vi "Translator.File.Read.FP.vi"(4 "progressbar2":refnum<vi>, 5 "init":bool, 6 "progressbar1":refnum<vi>, 7 "Message":refnum<vi>, 8 "error in":errorcluster, 9 "font name":string, 11 "Translation file":path=path "D:/PL_0125_Sapphire_Automation_branches/SOFTWARE_v1.1-Translation/settings/Translation-Chinese.ini") -> (0 "error out":errorcluster)   [LabVIEW 2016]
uses:
  Translator.Message.ctl
  Translator.Control.Fglb.Action.vi
  Translator.FormatMessage.vi
  Translator.Global.vi
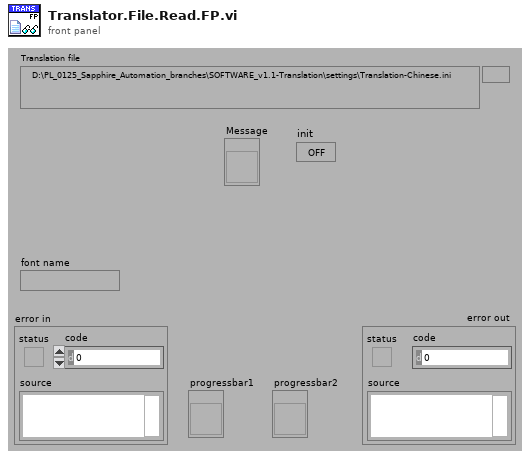
[diagram p1: front panel]
types:
  T1 = typedef "Translator.Message.ctl" = enum16{"-", "Event confirmed", "Log out", "Log in", "Shutdown", "Cancel", "Start", "Begin time", "End time", "Duration", "Service Mode", "Ignore Results", "Serial Format", "On", "Off", "OK", "NOK", "NOK %s", "Home", "Work", "Close", "Open", "In progress...", "Missing", "Empty", "Hardware failure", "Initial", "Default", "Total", "Out of range", "Free disk space is below 1GB - contact technician", "Error %d >> %s", "Error %d >> %s >> %s", "Msg %d >> %s", "Laser msg %d %s", "Laser cmd error %s %d", "Laser cmd failed %s", "Laser cmd warning %s", "Laser disconnected", "Laser status %s", "Laser already started", "Laser job unkonwn %s", "Laser job missing %s", "Laser job select failure %s", "Unable to start laser printing (%s)", "Unable to stop laser printing (%s)", "Laser marking aborted", "Laser marking timeout", "Unable to reset Laser Interlock (%s)", "Unable to trigger Laser. Laser not ready (%s)", "Laser job '%s' coordinates not configured", "Starting %s", "Quitting %s", "Configured", "Initializing", "Quitting", "Loading", "Loaded %d results", "Loaded %d events", "Running", "Stopped", "Summary", "Laser", "Do you want to continue?", "Do you want to delete the configuration?", "The configuration is being used by an order. Unable to delete!", "Press confirm button", "Station is not based. Do you want to exit?", "Station requires changeover. Do you want to run the test?", "Test options are not set as default. Do you want to continue?", "Formatting of WabcoNo is disabled. Do you want to continue?", "Product not detected. Do you want to continue?", "Product scan failed. Do you want to continue?", "Calibration", "Log out?", "System", "All", "IDLE", "Translating...%s", "Not found", "Alarm %s", "Run", "Skip", "Abort", "Repeat", "Please wait...", "Database disconnected", "Database disconnected - changeover disabled!", "Login to database successful", "Login to database failed: %d; %s", "Unable to check the product status of reference %d - database disconnected", "Unable to set the product status of reference %d - database disconnected", "Variant file backup %s", "Read variant (%s)", "Result", "Station armed!", "Station requires changeover!", "Select reference number...", "EMERGENCY BUTTON - press Control button", "EMERGENCY DOOR - press Control button", "Resetting Emergency...", "Unable to reset safety circuit - Emergency Button pressed", "Unable to reset safety circuit - Emergency Side Door open", "Station not based", "Station based", "Station not empty", "Station basing...", "No order", "Press Start to begin new order", "Scanning new order", "Order NOK. Correct or scan again", "Order OK. Press Accept", "Order ready", "Revolver incorrect", "Fork incorrect", "Revolver missing", "Revolver empty", "Container missing", "Offline results", "Offline statistics", "Updating statistics %.1f %%", "DMC Configurator", "Door open", "Close the front door", "Press start button", "Done. Open the front door", "Running...", "Running...%.1f %%", "Pause %s", "Pause %s. NOK container missing", "Pause %s. OK container missing", "Pause %s. Revolver empty", "Pause %s. Revolver missing", "Pause %s. Revolver incorrect", "Pause %s. Fork missing", "Pause %s. Fork incorrect", "Pause %s. Too many failures", "Pause %s. Unloading failure", "Pause %s. One slot is not working", "Pause %s. Part order is done. Empty OK container", "Pause %s. Unable to move product to slot", "Pause %s. Unable to move back product pusher", "Pause %s. Unable to lift product", "Pause %s. Unable to move back product lifter", "Pause %s. Unable to move product arm to Work", "Pause %s. Unable to move product arm to NOK", "Pause %s. Unable to move product arm to OK", "Pause %s. Unable to unsuck the NOK product", "Pause %s. Unable to drop the NOK product", "Pause %s. Product OK missing", "Pause %s. Unable to unsuck the OK product", "Pause %s. Unable to drop the OK product", "Stopping...", "File '%s' is missing", "File '%s' is broken", "File '%s' is running", "Log file started (%s)", "Log file ended (%s)", "Log file stopped (%s)", "Log file ignored (%s)", "Log file exported (%s)", "Log file export failed (%s)", "Wrong serial number in log file", "Wrong reference number in log file", "Test steps are missing", "%s = %.3f", "Process param '%s' not found in DB", "Process param '%s' wrong order", "Process param '%s' value %.3f out of limits (%.3f; %.3f)", "Step%d param '%s' not found in DB", "Step%d param '%s' wrong order", "Step%d param '%s' value %.3f out of limits (%.3f; %.3f)", "Step%d EV '%s' not found in DB", "Step%d EV '%s' wrong order", "\"%s\" not found in DB", "\"%s\" wrong order", "\"%s\" value %.3f out of limits (%.3f; %.3f)", "\"%s\" not found in software", "Process init (%s)", "Process started", "Process restarted", "Process run", "Process done", "Process done - remove OK container", "Process aborted", "Process aborted at work", "Process aborted at home", "Process error", "Process error at home", "Process error at work", "Process close", "Process pause", "Process continue", "Process door open", "Process door close", "Process pause at slot %s due to %s", "Select plate from the order to process", "Do you want to start the process?", "Do you want to continue the process?", "There is unfinished order. Do you want to put the new order?", "Product %s %d OK", "Product %s %d NOK", "Unable to unload the slot %s. Product missing in the slot", "Unable to unload the slot %s. Product already in the arm", "Unable to accept the product as OK. Product missing in slot %s", "Unable to accept the product as OK. Product could not drop into the container at slot %s", "Unable to accept the product as NOK. Product could not drop into the container at slot %s", "Scan failed. Error %s", "Scan failed. Scanner disconnected", "Scan failed. Wrong Wabco number %d, limit (%d,%d)", "Scan failed. Wrong serial number %d, limit (%d,%d)", "Scan failed. Wrong date %d, limit (%d,%d)", "Scan failed. Wrong product wabco number %d (expected %d)", "Scan failed. Wrong product serial number %d (expected > 0)", "Scan OK %s", "Scan failed. Unable to determine table position (%s)", "Scan failed. Timeout", "Tune failed. Scanner disconnected", "Tune failed. Timeout", "%s = %d", "%s = %d->%d", "Unable to set %s = %.2f - Air Pressure Inside off", "Unable to set digital output '%s' = %d", "Unable to activate air pressure inside - timeout", "Unable to activate air pressure inside - aborted", "Unable to switch on Air Main Valve - Air Pressure Inlet off", "Unable to switch on Air Main Valve - Door open", "Unable to switch off Air Main Valve - timeout", "Unable to switch off Air Main Valve - aborted", "Unable to rotate Table - timeout", "Unable to rotate Table - aborted", "Unable to rotate Table - Product Move not in Home position", "Unable to rotate Table - Air Pressure Inside off", "Unable to rotate Table - Product Lift A not in Home position", "Unable to rotate Table - Product Lift B not in Home position", "Unable to rotate Table - unlock before movement timeout", "Unable to rotate Table - lock after movement timeout", "Unable to move Table Lock to %s position - timeout", "Unable to move Table Lock to %s position - aborted", "Unable to move Table Lock to %s position - Air Pressure Inside off", "Unable to move Table Lock to %s position - Table not in position", "Unable to move Product Lift A to %s position - timeout", "Unable to move Product Lift B to %s position - timeout", "Unable to move Product Lift A to %s position - aborted", "Unable to move Product Lift B to %s position - aborted", "Unable to move Product Lift A to %s position - Air Pressure Inside off", "Unable to move Product Lift B to %s position - Air Pressure Inside off", "Unable to move Product Lift A to %s position - Table not locked", "Unable to move Product Lift B to %s position - Table not locked", "Unable to move Product Lift A to %s position - Product Arm not in Work position", "Unable to move Product Lift B to %s position - Product Arm not in Work position", "Unable to set Product Suction Gripper %s to %s - timeout", "Unable to set Product Suction Gripper %s to %s - aborted", "Unable to set Product Suction Gripper %s to %s - Air Pressure Inside off", "Unable to set Product Suction Gripper %s to %s - Table slot unkown", "Unable to move Product Arm to %s position - timeout", "Unable to move Product Arm to %s position - aborted", "Unable to move Product Arm to %s position - Air Pressure Inside off", "Unable to move Product Arm to %s position - Product Lift A not in Home position", "Unable to move Product Arm to %s position - Product Lift B not in Home position", "Unable to move Product to %s position - timeout", "Unable to move Product to %s position - aborted", "Unable to move Product to %s position - Air Pressure Inside off", "Unable to move Product to %s position - Table not in position"}
  T2 = typedef "Translator.Control.Fglb.Action.vi" = enum16{"init", "set", "get", "clear"}
  T3 = typedef "Translator.ControlData.ctl" = cluster{"ref":refnum<vi>, "strict?":bool, "save font?":bool, "type":T4, "root":string, "label":string, "caption":string, "bln.false":string, "bln.true":string, "cols":string[], "rows":string[]}
  T4 = typedef "Translator.ControlTypes.ctl" = enum16{"Cluster", "Array", "Boolean", "Ring", "String", "Tab", "Listbox", "Multicolumn listbox", "Table", "Tree", "Other"}
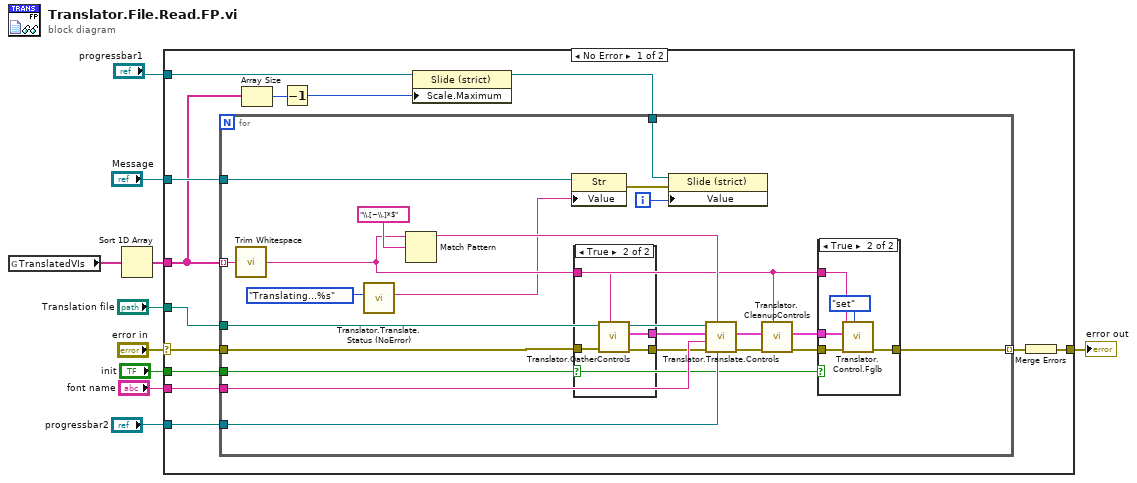
[diagram p0: block diagram]
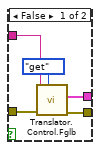
[diagram p3: hidden frame]
diagram:
  n1 = global read "Translator.Global.vi" "TranslatedVIs"() -> (w2:string[])
  n2 = Sort 1D Array(array=w2) -> (sorted array=w3:string[])
  n3 = case shown="No Error" "error in" {
    selector: "error in" -> [w22 w59]
    tunnel: "Translation file" -> [w20 _]
    tunnel: [w12 w59] -> w9
    tunnel: w3 -> [w15 _]
    tunnel: "font name" -> [w23 _]
    tunnel: "progressbar2" -> [w19 _]
    tunnel: "Message" -> [w18 _]
    tunnel: "progressbar1" -> [w14 _]
    tunnel: "init" -> [w11 _]
    frame No Error {
      n4 = Array Size(array=w15) -> (size(s)=w17:i32)
      n5 = Decrement(x=w17) -> (x-1=w16:i32)
      n6 = property on="Property Node" class="Slide (strict)"(reference=w14, "Scale.Maximum"=w16) -> (reference out=w13:refnum<vi>)  [unwired: 1 in, 1 out]
      n7 = for {
        tunnel: w15 -> [w42] mode=indexing
        tunnel: w23 -> [w43]
        tunnel: w20 -> [w37]
        tunnel: w19 -> [w41]
        tunnel: w18 -> [w40]
        tunnel: w13 -> [w39]
        tunnel: w22 -> [w24]
        tunnel: [w27] -> w21 mode=indexing
        tunnel: w11 -> [w36]
        i -> [w38]
        n8 = call <vilib>:"Trim Whitespace.vi"("string"=w42) -> ("trimmed string"=w28:string)  [unwired: 1 in]
        n9 = call "Translator.Translate.Status (NoError).vi"("msg"=Translator.Message."Translating...%s") -> ("Translated Msg"=w25:string)  [unwired: 10 in]
        n10 = Match Pattern(string=w28, regular expression="\\.[~\\.]*$") -> (before substring=w31:string)  [unwired: 4 out]
        n11 = property class="Str"(reference=w40, "Value"=w25) -> (error out=w33:errorcluster)  [unwired: 1 in, 1 out]
        n12 = case shown="True" w36 {
          tunnel: [w53 w58] -> w35
          tunnel: w24 -> [w52 w57]
          tunnel: [w51 w56] -> w30
          tunnel: w28 -> [w50 w55]
          frame False {
            n13 = call "Translator.Control.Fglb.vi"("Action"=Translator.Control.Fglb.Action.vi."get", "error in (no error)"=w52, "VI name"=w50) -> ("error out"=w53:errorcluster, "Controls out"=w51:T3[])  [unwired: 7 in]
          }
          frame True {
            n14 = call "Translator.GatherControls.vi"("VI name"=w55, "error in"=w57) -> ("error out"=w58:errorcluster, "Controls out"=w56:T3[])  [unwired: 8 in]
          }
        }
        n15 = property on="Property Node" class="Slide (strict)"(reference=w39, error in=w33, "Value"=w38) -> ()  [unwired: 2 out]
        n16 = call "Translator.Translate.Controls.vi"("progressbar"=w41, "group"=w31, "error in"=w35, "font name"=w43, "Controls out"=w30, "Translation file"=w37) -> ("error out"=w34:errorcluster)  [unwired: 5 in]
        n17 = call "Translator.CleanupControls.vi"("VI name"=w28, "error in"=w34, "Controls"=w30) -> ("error out"=w29:errorcluster)  [unwired: 8 in]
        n18 = case shown="True" w36 {
          tunnel: w30 -> [_ w49]
          tunnel: w28 -> [_ w48]
          tunnel: w29 -> [w44 w46]
          tunnel: [w44 w45] -> w27
          frame False {
          }
          frame True {
            n19 = call "Translator.Control.Fglb.vi"("Action"=Translator.Control.Fglb.Action.vi."set", "error in (no error)"=w46, "Controls in"=w49, "VI name"=w48) -> ("error out"=w45:errorcluster)  [unwired: 6 in, 1 out]
          }
        }
      }
      n20 = Merge Errors(w21) -> (w12:errorcluster)
    }
    frame Error {
    }
  }
  "error out" <- w9
